vi "PH_PP_CurrentMeas.evt call Select PA and FR.vi"(0 "i ref in":refnum<vi>, 2 "Instance name":string, 3 "Select PA/FR":bool, 5 "error in (no error)":errorcluster) -> (14 "i ref out":refnum<vi>, 19 "error out":errorcluster)   [LabVIEW 2014, in "PH_PP_CurrentMeas.lvlib"]
doc: "This VI calls an event by a simple call."
uses:
  PH_PP_CurrentMeas.lvlib
  CSCore/CSSystem/CoreLib/CoreLib.short 2 byte array.vi
  CSCore/BaseProcess/BaseProcess.lvlib
  CSCore/CSSystem/CoreLib/CoreLib.lvlib
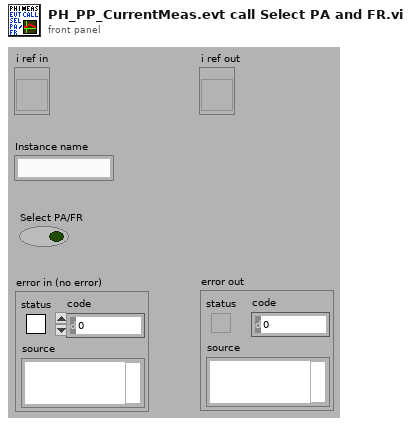
[diagram p1: front panel]
types:
  T1 = typedef "CoreDefs.rawDataType.ctl" = i8[]
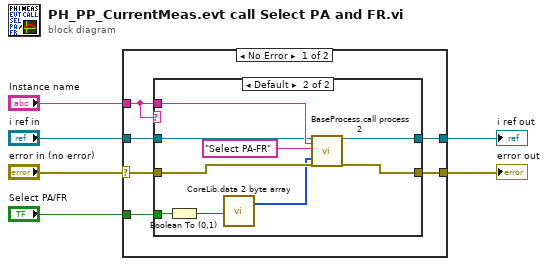
[diagram p0: block diagram]
diagram:
  n1 = case shown="No Error" "error in (no error)" {
    selector: "error in (no error)" -> [w7 w24]
    tunnel: "Select PA/FR" -> [w12 _]
    tunnel: "Instance name" -> [w8 _]
    tunnel: "i ref in" -> [w11 w25]
    tunnel: [w10 w25] -> w3
    tunnel: [w9 w24] -> w2
    frame No Error {
      n2 = case shown="Default" w8 {
        tunnel: w12 -> [_ w17]
        tunnel: w8 -> [_ w22]
        tunnel: w7 -> [w13 w21]
        tunnel: w11 -> [w14 w20]
        tunnel: [w14 w19] -> w10
        tunnel: [w13 w18] -> w9
        frame "N/A" {
        }
        frame Default {
          n3 = Boolean To (0,1)(Boolean=w17) -> (0, 1=w16:i16)
          n4 = call-poly "CoreLib.data 2 byte array.vi"("i16"=w16) -> ("byteArray out"=w15:T1)  [unwired: 18 in]
          n5 = call "BaseProcess.call process 2.vi"("i ref in"=w20, "Object"=w22, "Selector"="Select PA-FR", "Data"=w15, "error in (no error)"=w21) -> ("i ref out"=w19:refnum<vi>, "error out"=w18:errorcluster)  [unwired: 13 in]
        }
      }
    }
    frame Error {
    }
  }
  "error out" <- w2
  "i ref out" <- w3
